vi "paraCfgRowFormatChk.vi"(8 "error in":errorcluster, 9 "Row number":u32, 10 "Tbl Refnum in":refnum<vi>, 11 "Tree Refnum in":refnum<vi>) -> (0 "error out":errorcluster, 1 "chkRes":string="√", 2 "Tbl Refnum out":refnum<vi>, 3 "Tree Refnum out":refnum<vi>)   [LabVIEW 2010]
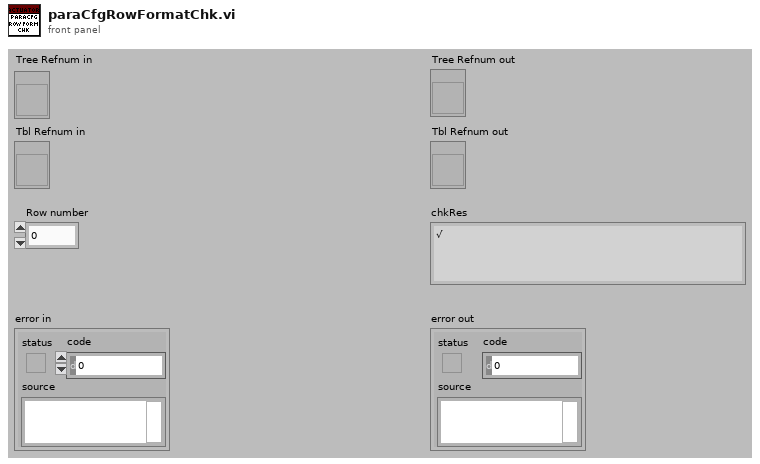
[diagram p1: front panel]
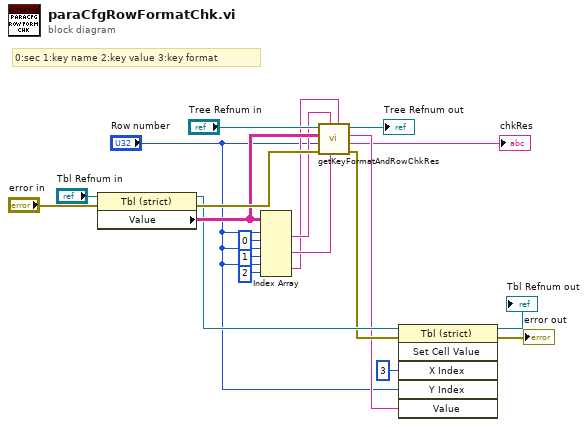
[diagram p0: block diagram]
diagram:
  # "0:sec 1:key name 2:key value 3:key format"
  n1 = property class="Tbl (strict)"(reference="Tbl Refnum in", error in="error in") -> (reference out=w9:refnum<vi>, error out=w17:errorcluster, "Value"=w16:string[][])
  n2 = Index Array(array=w16, index (row) #1="Row number", index (col) #1=0 ("index (row)"), index (row) #2="Row number", index (col) #2=1 ("disabled index (col)"), index (row) #3="Row number", index (col) #3=2 ("disabled index (col)")) -> (element #1=w12:string, element #2=w11:string, element #3=w10:string)
  n3 = call "getKeyFormatAndRowChkRes.vi"("keyVal"=w10, "keyName"=w11, "section"=w12, "error in"=w17, "Row number"="Row number", "table"=w16, "Tree Refnum in"="Tree Refnum in") -> ("error out"=w8:errorcluster, "chkRes"=→"chkRes":string, "keyFormat"=w7:string, "Tree Refnum out"=→"Tree Refnum out":refnum<vi>)  [unwired: 1 in]
  n4 = invoke class="Tbl (strict)" method="Set Cell Value"(reference=w9, error in=w8, "X Index"=u32 3, "Y Index"="Row number", "Value"=w7) -> (reference out=→"Tbl Refnum out":refnum<vi>, error out=→"error out":errorcluster)  [unwired: 1 in, 4 out]
